vi "RX-BPCS-SIM-UDP.vi"(11 "Stop":bool) -> ()   [LabVIEW 2018]
uses:
  <vilib>/Platform/TimedLoop/XDataNode/timing_clust.ctl
  <vilib>/Platform/TimedLoop/XDataNode/nitl_modes.ctl
  <vilib>/Platform/TimedLoop/XDataNode/wakeup.ctl
  Global Variable.vi
  <vilib>/Platform/TimedLoop/XDataNode/XDataNode.xnode
  <vilib>/Platform/TimedLoop/XDataNode/XDNodeRunTimeDep.lvlib
panel:
  out "SIM-BPCS-RX-ARRAY":dbl[](array[numeric])
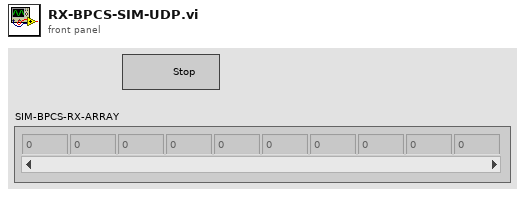
[diagram p1: front panel]
types:
  T1 = typedef "XDNodeRunTimeDep.lvlib/timing_clust.ctl" = cluster{"Expected End [f-1]":u64, "Actual End [f-1]":u64, "Finished Late? [f-1]":bool, "Expected End [i-1]":u64, "Actual End [i-1]":u64, "Finished Late? [i-1]":bool, "Expected Start [i]":u64, "Actual Start [i]":u64, "Expected Start [f]":u64, "Actual Start [f]":u64, "Source Name":string, "Structure Name":string, "Period":i64, "Deadline":i64, "Offset":i64, "Start":i64, "Priority":i32, "Timeout":i32, "Mode":T2, "Wakeup Reason":T3, "Error":errorcluster, "Source Type":string, "Secondary Source Type":string, "Global End Time":u64, "Global Start Time":u64, "Frame Duration":u64, "Iteration Duration":u64, "Assigned CPU":i32, "I/O Scan Engine Mode":u32}
  T2 = typedef "XDNodeRunTimeDep.lvlib/nitl_modes.ctl" = enum32{"No Change", "Process missed periods, maintain original phase", "Discard missed periods, maintain original phase", "Process missed periods, ignore original phase", "Discard missed periods, ignore original phase"}
  T3 = typedef "XDNodeRunTimeDep.lvlib/wakeup.ctl" = enum32{"Normal", "Aborted", "Asynchronous wakeup", "Timing source error", "Timed loop error", "Timeout"}
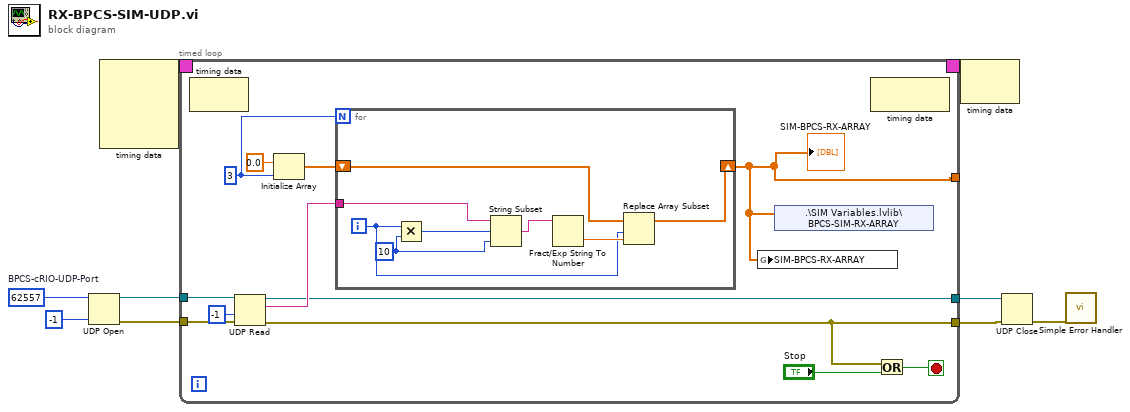
[diagram p0: block diagram]
diagram:
  w7 = u16 62557  # BPCS-cRIO-UDP-Port
  n1 = UDP Open(9:-1 ("timeout ms (25000)"), 11:w7) -> (port=w6:refnum<k16>, 0:w5:errorcluster)  [unwired: 3 in, 1 out]
  n2 = node-c288() -> (w9:T1)  [unwired: 4 in]
  n3 = timed-loop {
    timing: w9 -> [_]
    timing-out: [_] -> w8
    tunnel: w6 -> [w19]
    tunnel: w5 -> [w18]
    tunnel: [w16] -> w3
    tunnel: [w15] -> w2
    tunnel: [w10] -> _
    stop <- w20 stop-if-true
    w12 = 3 ("dimension size")
    n4 = node-c288() -> ()  [unwired: 1 in, 1 out]
    n5 = UDP Read(connection ID=w19, timeout ms (25000)=-1, 8:w18) -> (data out=w17:string, error out=w15:errorcluster, 3:w16:refnum<k16>)  [unwired: 3 out]
    n6 = Initialize Array(0.0 ("element"), w12) -> (w13:dbl[])
    n7 = for {
      N: w12 -> [_]
      tunnel: w17 -> [w28]
      shift-right: [w24] -> w10
      shift-left: w13 -> [w23]
      i -> [w25]
      w22 = 10 ("y")
      n8 = Multiply(x=w25, y=w22) -> (x*y=w27:i32)
      n9 = String Subset(string=w28, offset (0)=w27, length (rest)=w22) -> (substring=w29:string)
      n10 = Fract/Exp String To Number(string=w29) -> (number=w26:dbl)  [unwired: 3 in, 1 out]
      n11 = Replace Array Subset(array=w23, new element=w26, index=w25) -> (w24:dbl[])
    }
    "SIM-BPCS-RX-ARRAY" <- w10
    n12 = global write "Global Variable.vi" "SIM-BPCS-RX-ARRAY"(w10) -> ()
    n13 = shared-variable ".\\SIM Variables.lvlib\\BPCS-SIM-RX-ARRAY"(w10) -> ()  [unwired: 1 in, 1 out]
    n14 = node-c288() -> ()  [unwired: 1 in, 1 out]
    n15 = Or(x=w15, y="Stop") -> (x .or. y?=w20:bool)
  }
  n16 = node-c288(w8) -> ()  [unwired: 1 out]
  n17 = UDP Close(connection ID=w3, 8:w2) -> (error out=w4:errorcluster)  [unwired: 1 out]
  n18 = call <vilib>:"Simple Error Handler.vi"("error in (no error)"=w4) -> ()  [unwired: 4 in, 5 out]
